vi "Indexer.vi"(11 "Robot Commands":T1) -> ()   [LabVIEW 2015]
uses:
  Joystick/Robot Commands.ctl
  <vilib>/Rock Robotics/WPI/Relay/WPI_RelayValue.ctl
  Global Variables/Refnum Names.vi
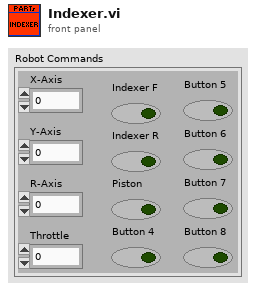
[diagram p1: front panel]
types:
  T1 = typedef "Robot Commands.ctl" = cluster{"X-Axis":dbl, "Y-Axis":dbl, "R-Axis":dbl, "Throttle":dbl, "Indexer F":bool, "Indexer R":bool, "Piston":bool, "Button 4":bool, "Button 5":bool, "Button 6":bool, "Button 7":bool, "Button 8":bool}
  T2 = typedef "WPI_RelayValue.ctl" = enum16{"Off", "On", "Forward", "Reverse"}
  T3 = typedef "WPI_RelayDevRef.ctl" = cluster{"DevStatus":errorcluster, "Relay Channel":T4, "Relay Direction":T5}
  T4 = typedef "FPGA_DIORelayChannel.ctl" = enum8{"Relay 0", "Relay 1", "Relay 2", "Relay 3", "Invalid"}
  T5 = typedef "WPI_RelayDirection.ctl" = enum16{"Both directions", "Forward only", "Reverse only"}
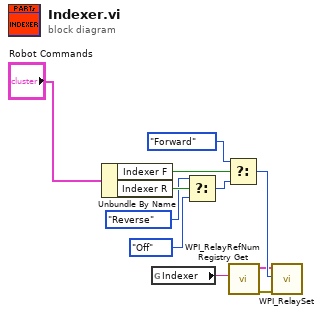
[diagram p0: block diagram]
diagram:
  n1 = Unbundle By Name("Robot Commands") -> ("Indexer F"=w6:bool, "Indexer R"=w4:bool)
  n2 = global read "Refnum Names.vi" "Indexer"() -> (w11:string)
  n3 = Select(t=WPI_RelayValue."Reverse" ("RelayValue"), s=w4, f=WPI_RelayValue."Off" ("RelayValue")) -> (s? t:f=w2:T2)
  n4 = Select(t=WPI_RelayValue."Forward" ("RelayValue"), s=w6, f=w2) -> (s? t:f=w10:T2)
  n5 = call <vilib>:"WPI_RelayRefNum Registry Get.vi"("refnum name"=w11) -> ("error out"=w9:errorcluster, "RelayDevRef"=w8:T3)  [unwired: 9 in]
  n6 = call <vilib>:"WPI_RelaySet.vi"("error in (no error)"=w9, "RelayValue"=w10, "RelayDevRef"=w8) -> ()  [unwired: 7 in, 2 out]
